vi "Shutdown.vi"(8 "error in":errorcluster, 11 "Framework Engine.lvclass":refnum<class "Framework Engine.lvclass">) -> (0 "error out":errorcluster, 3 "output cluster":refnum<class "Framework Engine.lvclass">)   [LabVIEW 2026, in "Framework Engine.lvclass"]
uses:
  Framework Engine.lvclass
  Framework Engine.lvclass/Framework Engine.ctl
  Domain/Session/Session.lvclass
  Domain/User/User.lvclass
  Services/Authentication Service/Authentication Service.lvclass
  Services/Execution Service/Execution Service.lvclass
  Services/Logging Service/Logging Service.lvclass
  Services/Readiness Service/Readines Service.lvclass
  Services/Settings Service/Settings Service.lvclass
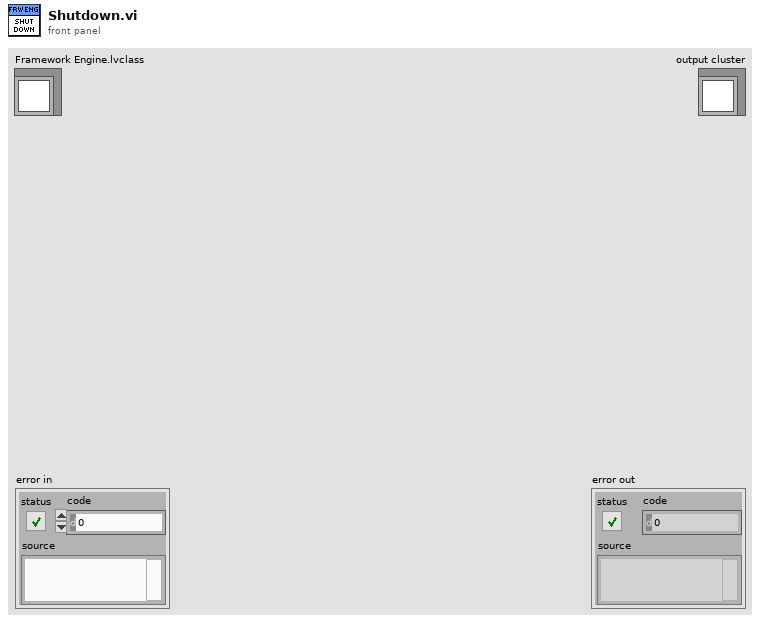
[diagram p1: front panel]
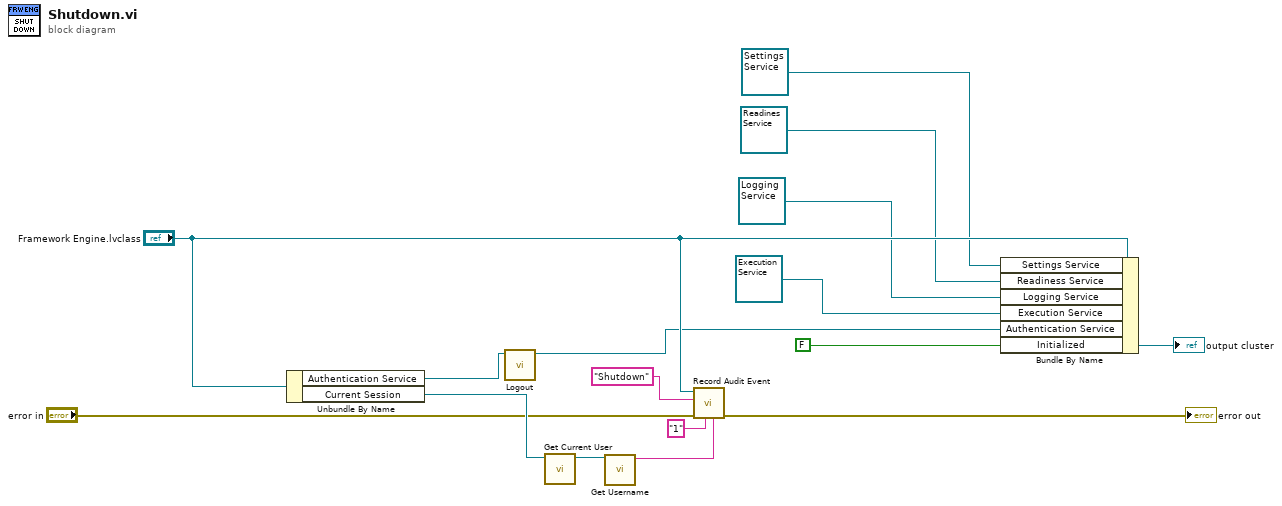
[diagram p0: block diagram]
diagram:
  n1 = Unbundle By Name("Framework Engine.lvclass") -> ("Authentication Service"=w6:refnum<class "Authentication Service.lvclass">, "Current Session"=w16:refnum<class "Session.lvclass">)
  n2 = call "Logout.vi"("Authentication Service in"=w6) -> ("Authentication Service out"=w5:refnum<class "Authentication Service.lvclass">)  [unwired: 10 in]
  n3 = call "Get Current User.vi"("Session Data"=w16) -> ("Current User"=w15:refnum<class "User.lvclass">)  [unwired: 10 in]
  n4 = call "Get Username.vi"("User Data"=w15) -> ("Username"=w14:string)  [unwired: 10 in]
  n5 = call "Record Audit Event.vi"("User"=w14, "Level"="1", "error in"="error in", "Message"="Shutdown", "Framework Engine in"="Framework Engine.lvclass") -> ("error out"=→"error out":errorcluster)  [unwired: 6 in]
  n6 = Bundle By Name(cluster="Framework Engine.lvclass", "Settings Service"=refnum<class "Settings Service.lvclass"> refnum, "Readiness Service"=refnum<class "Readines Service.lvclass"> refnum, "Logging Service"=refnum<class "Logging Service.lvclass"> refnum, "Execution Service"=refnum<class "Execution Service.lvclass"> refnum, "Authentication Service"=w5, "Initialized"=FALSE) -> (→"output cluster":refnum<class "Framework Engine.lvclass">)
